vi "Popup Menu Start.vi"(0 "VI Ref":refnum<vi>, 7 "Str Ctrl Ref":refnum<vi>, 9 "Initial Menu Options":string[](array[string]), 11 "Error In":errorcluster, 13 "XY Position":T1) -> (15 "Error Out":errorcluster)   [LabVIEW 2020]
uses:
  <vilib>/Utility/miscctls.llb/LVPointTypeDef.ctl
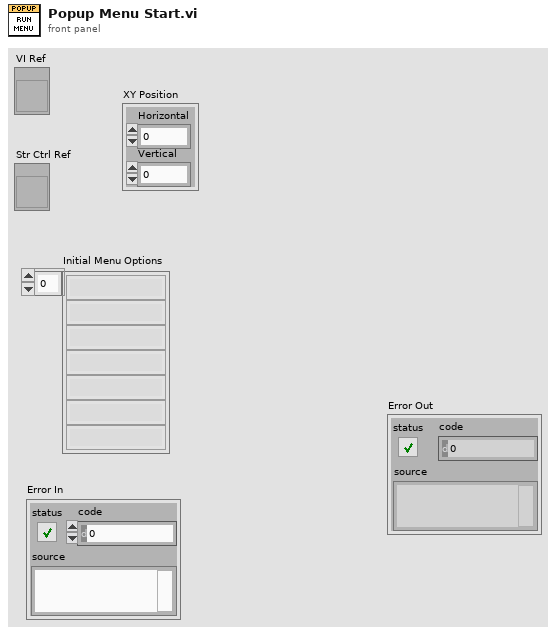
[diagram p1: front panel]
types:
  T1 = typedef "LVPointTypeDef.ctl" = cluster{"Horizontal":i16, "Vertical":i16}
  T2 = enum32{"Invalid", "Standard", "Closed", "Hidden", "Minimized", "Maximized"}
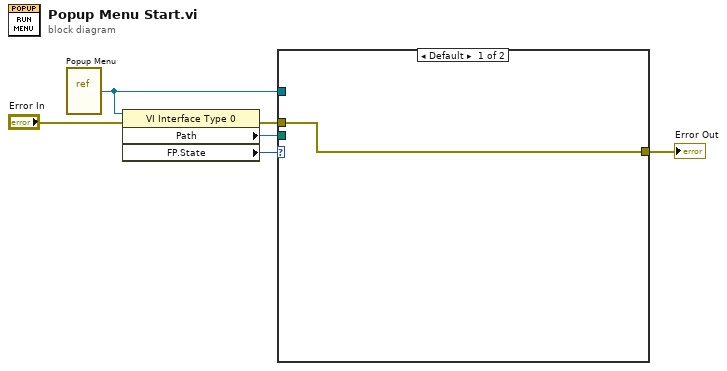
[diagram p0: block diagram]
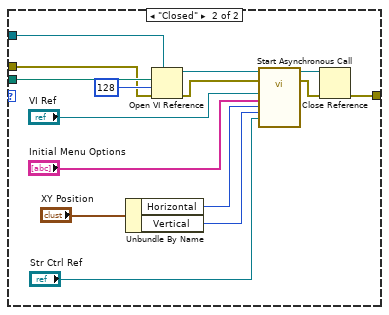
[diagram p2: hidden frame]
diagram:
  n1 = vi-ref "Popup Menu.vi"() -> (w6:refnum<vi>)
  n2 = property class="VI Interface Type 0"(reference=w6, error in="Error In") -> (error out=w3:errorcluster, "Path"=w5:path, "FP.State"=w4:T2)  [unwired: 1 out]
  n3 = case shown="Default" w4 {
    tunnel: w6 -> [_ w20]
    tunnel: w5 -> [_ w19]
    tunnel: w3 -> [w7 w11]
    tunnel: [w7 w8] -> w2
    frame Default {
    }
    frame "Closed" {
      n4 = Unbundle By Name("XY Position") -> ("Horizontal"=w15:i16, "Vertical"=w14:i16)
      n5 = Open VI Reference(type specifier VI Refnum (for type only)=w20, vi path=w19, options=128, error in (no error)=w11) -> (vi reference=w21:refnum<vi>, error out=w10:errorcluster)  [unwired: 2 in]
      n6 = call-by-ref "Start Asynchronous Call"(reference=w21, error in=w10, "Calling VI Ref"="VI Ref", "Initial Menu Options"="Initial Menu Options", "Left"=w15, "Top"=w14, "String Ctrl Ref"="Str Ctrl Ref") -> (reference out=w22:refnum<vi>, error out=w9:errorcluster)  [unwired: 10 in, 1 out]
      n7 = Close Reference(reference=w22, error in (no error)=w9) -> (error out=w8:errorcluster)
    }
  }
  "Error Out" <- w2
